vi "MFC Sequence File Check (SubVI).vi"(8 "error in (no error)":errorcluster, 10 "Sequence Cluster":T1(array[cluster]), 11 "Cluster of MFCs":T2(array[cluster])) -> (0 "error in (no error) 2":errorcluster)   [LabVIEW 2011]
uses:
  <vilib>/Utility/error.llb/DialogType.ctl
  Program Files (x86)/National Instruments/LabVIEW 2011/resource/objmgr/daqmx.rc
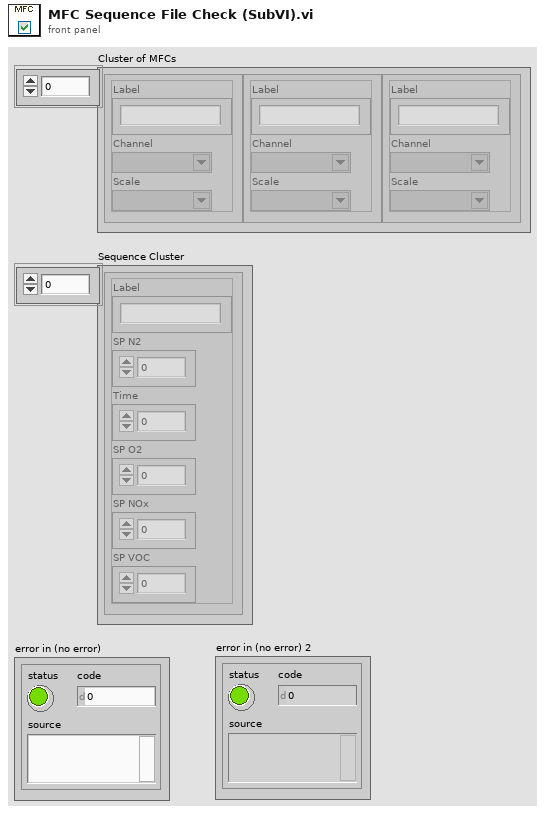
[diagram p1: front panel]
types:
  T1 = cluster{"Label":string, "SP N2":dbl, "Time":dbl, "SP O2":dbl, "SP NOx":dbl, "SP VOC":dbl}[]
  T2 = cluster{"Label":string, "Channel":tag, "Scale":tag}[]
  T3 = cluster{"Label":string, "Channel":tag, "Scale":tag}
  T4 = typedef "DialogType.ctl" = u16
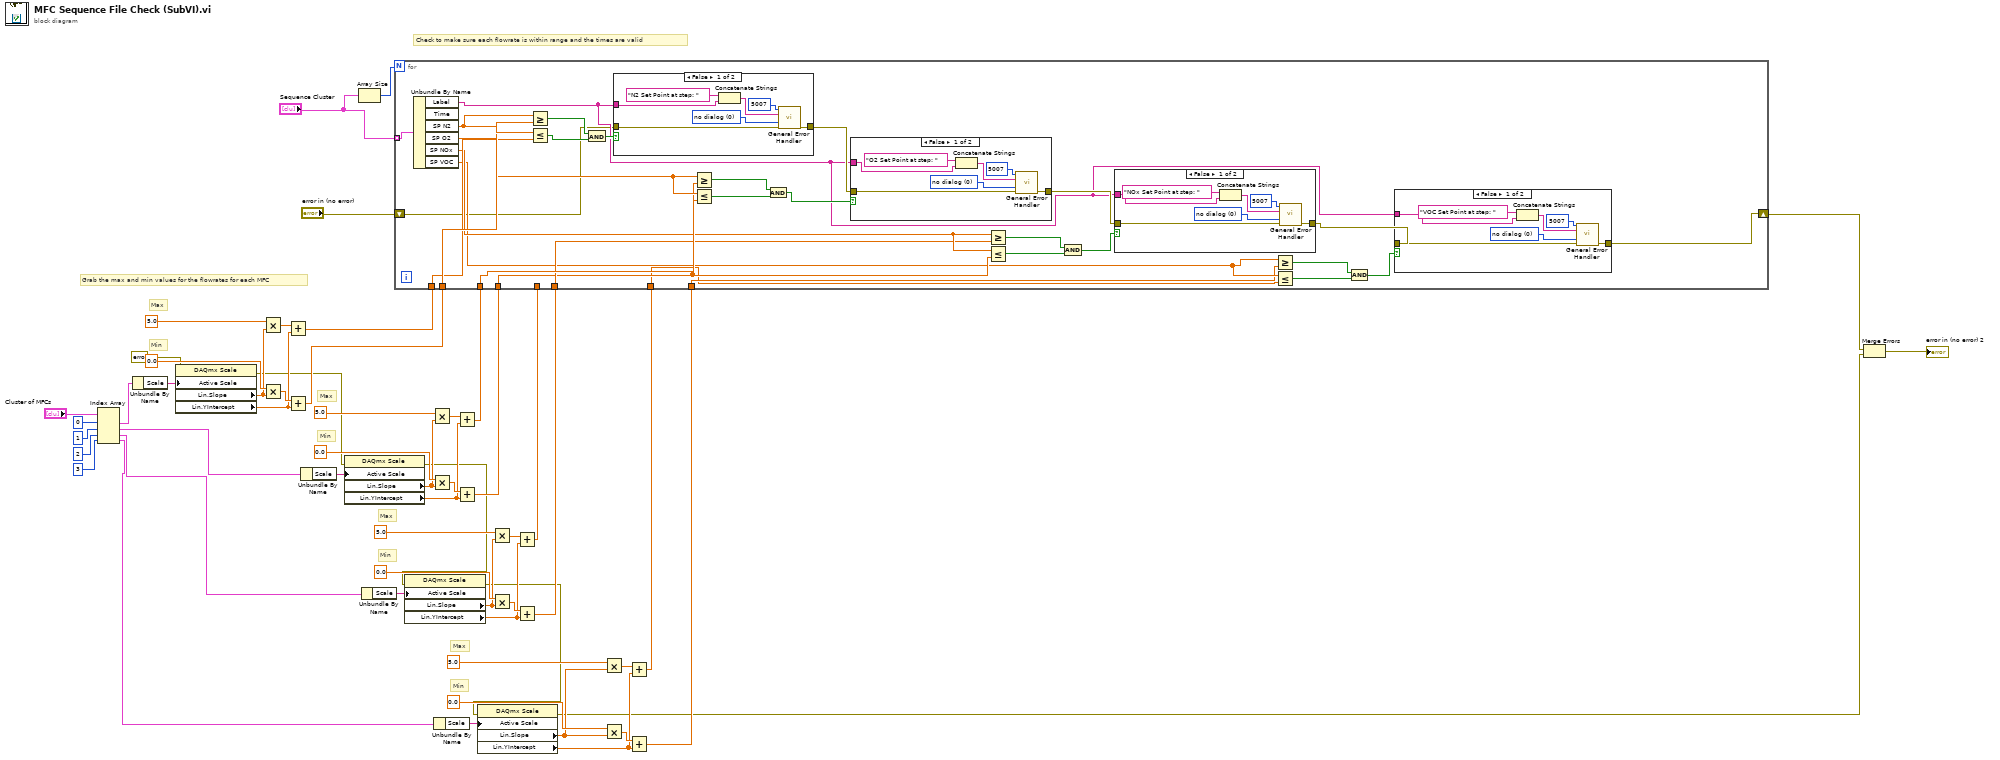
[diagram p0: block diagram]
diagram:
  # "Max"
  # "Min"
  # "Max"
  # "Min"
  # "Max"
  # "Min"
  # "Max"
  # "Min"
  # "Grab the max and min values for the flowrates for each MFC"
  # "Check to make sure each flowrate is within range and the times are valid"
  n1 = Index Array(array="Cluster of MFCs", index #1=0 ("index"), index #2=1 ("index"), index #3=2 ("index"), index #4=3 ("index")) -> (element #1=w48:T3, element #2=w33:T3, element #3=w21:T3, element #4=w11:T3)
  n2 = Unbundle By Name(w48) -> ("Scale"=w47:tag)
  n3 = property class="DAQmx Scale"(error in=errorcluster {"status"=FALSE, "code"=0, "source"=""} ("error in (no error)"), "Active Scale"=w47) -> (error out=w7:errorcluster, "Lin.Slope"=w42:dbl, "Lin.YIntercept"=w41:dbl)  [unwired: 1 in, 1 out]
  n4 = Multiply(x=5.0, y=w42) -> (x*y=w44:dbl)
  n5 = Multiply(x=0.0, y=w42) -> (x*y=w46:dbl)
  n6 = Add(x=w44, y=w41) -> (x+y=w32:dbl)
  n7 = Add(x=w46, y=w41) -> (x+y=w31:dbl)
  n8 = Unbundle By Name(w33) -> ("Scale"=w40:tag)
  n9 = property class="DAQmx Scale"(error in=w7, "Active Scale"=w40) -> (error out=w6:errorcluster, "Lin.Slope"=w35:dbl, "Lin.YIntercept"=w34:dbl)  [unwired: 1 in, 1 out]
  n10 = Array Size(array="Sequence Cluster") -> (size(s)=w54:i32)
  n11 = Unbundle By Name(w21) -> ("Scale"=w28:tag)
  n12 = property class="DAQmx Scale"(error in=w6, "Active Scale"=w28) -> (error out=w5:errorcluster, "Lin.Slope"=w23:dbl, "Lin.YIntercept"=w22:dbl)  [unwired: 1 in, 1 out]
  n13 = Multiply(x=5.0, y=w35) -> (x*y=w37:dbl)
  n14 = Multiply(x=0.0, y=w35) -> (x*y=w39:dbl)
  n15 = Unbundle By Name(w11) -> ("Scale"=w18:tag)
  n16 = Add(x=w37, y=w34) -> (x+y=w30:dbl)
  n17 = Add(x=w39, y=w34) -> (x+y=w29:dbl)
  n18 = property class="DAQmx Scale"(error in=w5, "Active Scale"=w18) -> (error out=w2:errorcluster, "Lin.Slope"=w13:dbl, "Lin.YIntercept"=w12:dbl)  [unwired: 1 in, 1 out]
  n19 = Multiply(x=5.0, y=w23) -> (x*y=w25:dbl)
  n20 = Multiply(x=0.0, y=w23) -> (x*y=w27:dbl)
  n21 = Add(x=w25, y=w22) -> (x+y=w20:dbl)
  n22 = Add(x=w27, y=w22) -> (x+y=w19:dbl)
  n23 = Multiply(x=5.0, y=w13) -> (x*y=w15:dbl)
  n24 = Multiply(x=0.0, y=w13) -> (x*y=w17:dbl)
  n25 = Add(x=w15, y=w12) -> (x+y=w10:dbl)
  n26 = Add(x=w17, y=w12) -> (x+y=w9:dbl)
  n27 = for {
    N: w54 -> [_]
    tunnel: "Sequence Cluster" -> [w85] mode=indexing
    shift-right: [w64] -> w3
    shift-left: "error in (no error)" -> [w56]
    tunnel: w32 -> [w82]
    tunnel: w31 -> [w83]
    tunnel: w30 -> [w73]
    tunnel: w29 -> [w66]
    tunnel: w20 -> [_]
    tunnel: w19 -> [w67]
    tunnel: w10 -> [w57]
    tunnel: w9 -> [w58]
    n28 = Unbundle By Name(w85) -> ("Label"=w63:string, "SP N2"=w84:dbl, "SP O2"=w74:dbl, "SP NOx"=w68:dbl, "SP VOC"=w59:dbl)  [unwired: 1 out]
    n29 = Greater Or Equal?(x=w84, y=w83) -> (x >= y?=w81:bool)
    n30 = Less Or Equal?(x=w84, y=w82) -> (x <= y?=w80:bool)
    n31 = And(x=w81, y=w80) -> (x .and. y?=w79:bool)
    n32 = case shown="False" w79 {
      tunnel: w56 -> [w116 w117]
      tunnel: [w115 w117] -> w78
      tunnel: w63 -> [w110 _]
      frame False {
        w113 = T4 0 items=["no dialog", "OK message", "continue or stop message", "OK message + warnings", "continue/stop + warnings"] ("type of dialog (OK msg:1)")
        n33 = Concatenate Strings("N2 Set Point at step: " ("[error source] (\" \")"), w110) -> (w112:string)
        n34 = call <vilib>:"General Error Handler.vi"("[error code] (0)"=5007, "[error source] (\" \")"=w112, "type of dialog (OK msg:1)"=w113, "error in (no error)"=w116) -> ("error out"=w115:errorcluster)  [unwired: 7 in, 4 out]
      }
      frame True {
      }
    }
    n35 = Greater Or Equal?(x=w74, y=w66) -> (x >= y?=w76:bool)
    n36 = Less Or Equal?(x=w74, y=w73) -> (x <= y?=w75:bool)
    n37 = And(x=w76, y=w75) -> (x .and. y?=w77:bool)
    n38 = case shown="False" w77 {
      tunnel: w78 -> [w108 w109]
      tunnel: [w107 w109] -> w72
      tunnel: w63 -> [w102 _]
      frame False {
        w105 = T4 0 items=["no dialog", "OK message", "continue or stop message", "OK message + warnings", "continue/stop + warnings"] ("type of dialog (OK msg:1)")
        n39 = Concatenate Strings("O2 Set Point at step: " ("[error source] (\" \")"), w102) -> (w104:string)
        n40 = call <vilib>:"General Error Handler.vi"("[error code] (0)"=5007, "[error source] (\" \")"=w104, "type of dialog (OK msg:1)"=w105, "error in (no error)"=w108) -> ("error out"=w107:errorcluster)  [unwired: 7 in, 4 out]
      }
      frame True {
      }
    }
    n41 = Greater Or Equal?(x=w68, y=w67) -> (x >= y?=w71:bool)
    n42 = Less Or Equal?(x=w68, y=w66) -> (x <= y?=w70:bool)
    n43 = And(x=w71, y=w70) -> (x .and. y?=w69:bool)
    n44 = case shown="False" w69 {
      tunnel: w72 -> [w100 w101]
      tunnel: [w99 w101] -> w65
      tunnel: w63 -> [w94 _]
      frame False {
        w97 = T4 0 items=["no dialog", "OK message", "continue or stop message", "OK message + warnings", "continue/stop + warnings"] ("type of dialog (OK msg:1)")
        n45 = Concatenate Strings("NOx Set Point at step: " ("[error source] (\" \")"), w94) -> (w96:string)
        n46 = call <vilib>:"General Error Handler.vi"("[error code] (0)"=5007, "[error source] (\" \")"=w96, "type of dialog (OK msg:1)"=w97, "error in (no error)"=w100) -> ("error out"=w99:errorcluster)  [unwired: 7 in, 4 out]
      }
      frame True {
      }
    }
    n47 = Greater Or Equal?(x=w59, y=w58) -> (x >= y?=w62:bool)
    n48 = Less Or Equal?(x=w59, y=w57) -> (x <= y?=w61:bool)
    n49 = And(x=w62, y=w61) -> (x .and. y?=w60:bool)
    n50 = case shown="False" w60 {
      tunnel: w65 -> [w92 w93]
      tunnel: [w91 w93] -> w64
      tunnel: w63 -> [w86 _]
      frame False {
        w89 = T4 0 items=["no dialog", "OK message", "continue or stop message", "OK message + warnings", "continue/stop + warnings"] ("type of dialog (OK msg:1)")
        n51 = Concatenate Strings("VOC Set Point at step: " ("[error source] (\" \")"), w86) -> (w88:string)
        n52 = call <vilib>:"General Error Handler.vi"("[error code] (0)"=5007, "[error source] (\" \")"=w88, "type of dialog (OK msg:1)"=w89, "error in (no error)"=w92) -> ("error out"=w91:errorcluster)  [unwired: 7 in, 4 out]
      }
      frame True {
      }
    }
  }
  n53 = Merge Errors(w3, w2) -> (→"error in (no error) 2":errorcluster)
